vi "CalcIMUBias.vi"(10 "error in (no error)":errorcluster) -> (1 "Bias":T1, 3 "error out":errorcluster)   [LabVIEW 2016]
uses:
  <vilib>/Platform/TimedLoop/XDataNode/timing_clust.ctl
  <vilib>/Platform/TimedLoop/XDataNode/nitl_modes.ctl
  <vilib>/Platform/TimedLoop/XDataNode/wakeup.ctl
  <vilib>/Platform/TimedLoop/XDataNode/XDataNode.xnode
  <vilib>/Platform/TimedLoop/XDataNode/XDNodeRunTimeDep.lvlib
panel:
  out "Z gyro bias":dbl
  out "Y gyro bias":dbl
  out "X gyro bias":dbl
  out "Z acc bias":dbl
  out "Y acc bias":dbl
  out "X acc bias":dbl
  out "Accel, Gyro":u16[](array[numeric])
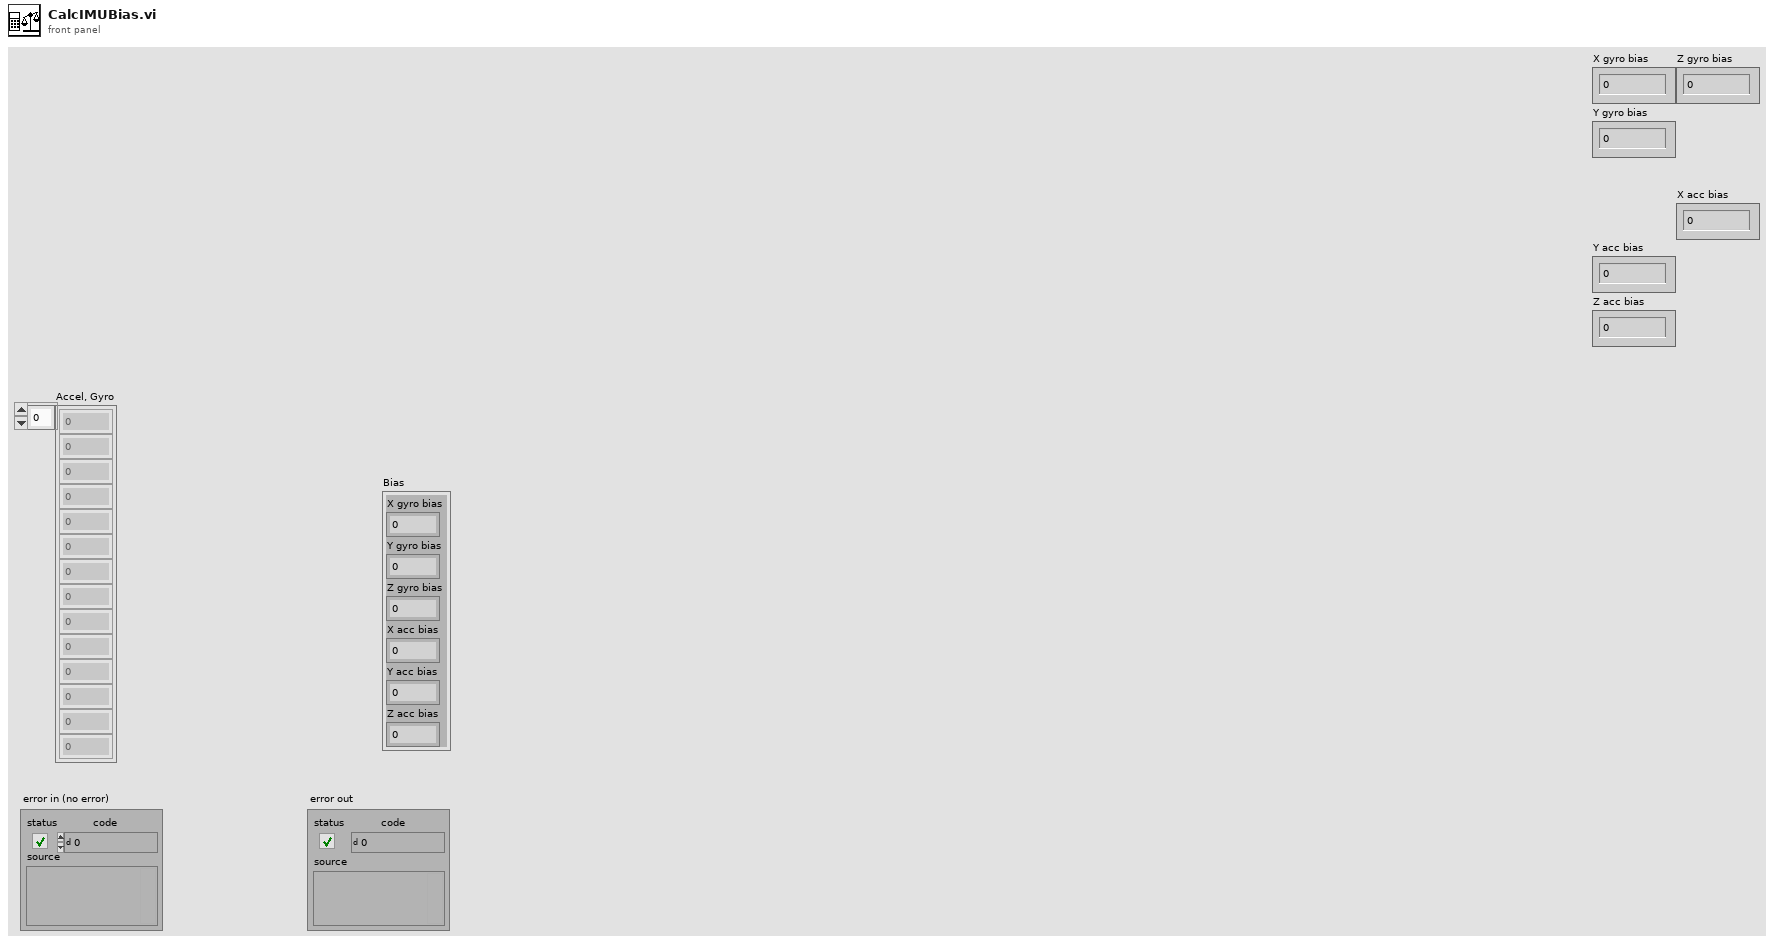
[diagram p1: front panel]
types:
  T1 = cluster{"X gyro bias":dbl, "Y gyro bias":dbl, "Z gyro bias":dbl, "X acc bias":dbl, "Y acc bias":dbl, "Z acc bias":dbl}
  T2 = typedef "XDNodeRunTimeDep.lvlib/timing_clust.ctl" = cluster{"Expected End [f-1]":u64, "Actual End [f-1]":u64, "Finished Late? [f-1]":bool, "Expected End [i-1]":u64, "Actual End [i-1]":u64, "Finished Late? [i-1]":bool, "Expected Start [i]":u64, "Actual Start [i]":u64, "Expected Start [f]":u64, "Actual Start [f]":u64, "Source Name":string, "Structure Name":string, "Period":i64, "Deadline":i64, "Offset":i64, "Start":i64, "Priority":i32, "Timeout":i32, "Mode":T3, "Wakeup Reason":T4, "Error":errorcluster, "Source Type":string, "Secondary Source Type":string, "Global End Time":u64, "Global Start Time":u64, "Frame Duration":u64, "Iteration Duration":u64, "Assigned CPU":i32, "I/O Scan Engine Mode":u32}
  T3 = typedef "XDNodeRunTimeDep.lvlib/nitl_modes.ctl" = enum32{"No Change", "Process missed periods, maintain original phase", "Discard missed periods, maintain original phase", "Process missed periods, ignore original phase", "Discard missed periods, ignore original phase"}
  T4 = typedef "XDNodeRunTimeDep.lvlib/wakeup.ctl" = enum32{"Normal", "Aborted", "Asynchronous wakeup", "Timing source error", "Timed loop error", "Timeout"}
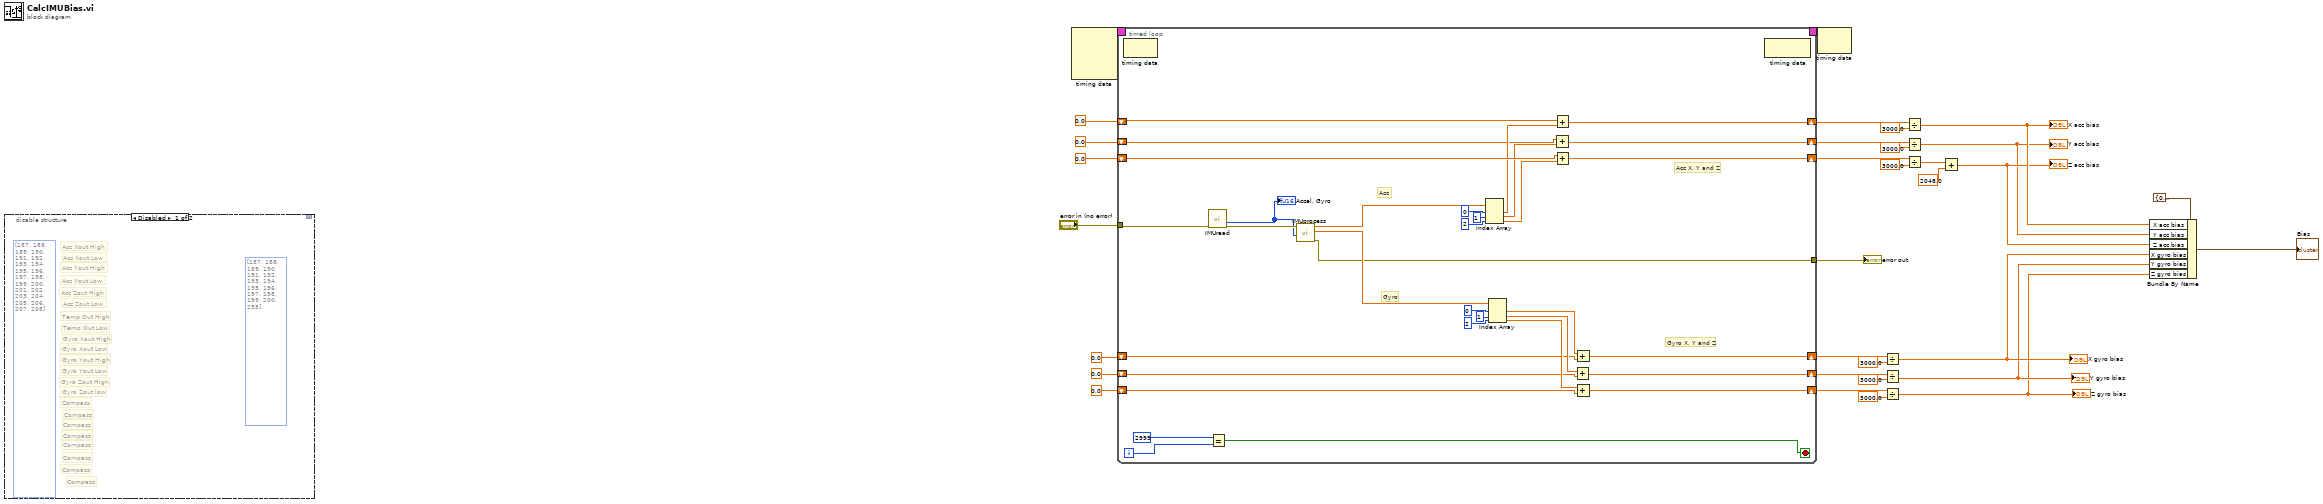
[diagram p0: block diagram]
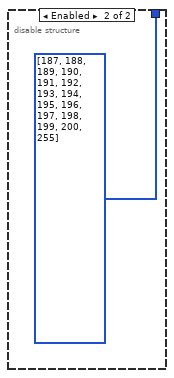
[diagram p2: hidden frame]
diagram:
  n1 = disable-structure shown="Disabled" {
    disable-tunnel: [_ u16[] [187, 188, 189, 190, 191, 192, 193, 194, 195, 196, 197, 198, 199, 200, 255] ("Frames to Write")] -> _
    frame Disabled {
      (unwired) u16[] [187, 188, 189, 190, 191, 192, 193, 194, 195, 196, 197, 198, 199, 200, 201, 202, 203, 204, 205, 206, 207, 208] ("Frames to Write")
      (unwired) u16[] [187, 188, 189, 190, 191, 192, 193, 194, 195, 196, 197, 198, 199, 200, 255] ("Frames to Write")
      # "Compass"
      # "Compass"
      # "Compass"
      # "Compass"
      # "Compass"
      # "Compass"
      # "Compass"
      # "Compass"
      # "Gyro Zout low"
      # "Gyro Zout High"
      # "Gyro Yout Low"
      # "Gyro Yout High"
      # "Gyro Xout Low"
      # "Gyro Xout High"
      # "Temp Out Low"
      # "Temp Out High"
      # "Acc Zout Low"
      # "Acc Zout High"
      # "Acc Yout Low"
      # "Acc Yout High"
      # "Acc Xout Low"
      # "Acc Xout High"
    }
    frame Enabled {
    }
  }
  n2 = node-c288() -> (w32:T2)  [unwired: 4 in]
  n3 = timed-loop {
    timing: w32 -> [_]
    timing-out: [_] -> w31
    shift-right: [w56] -> w22
    shift-left: 0.0 -> [w58]
    shift-right: [w55] -> w21
    shift-left: 0.0 -> [w52]
    shift-right: [w54] -> w20
    shift-left: 0.0 -> [w57]
    tunnel: [w49] -> w27
    tunnel: "error in (no error)" -> [w48]
    shift-right: [w47] -> w15
    shift-left: 0.0 -> [w41]
    shift-right: [w46] -> w14
    shift-left: 0.0 -> [w40]
    shift-right: [w45] -> w13
    shift-left: 0.0 -> [w39]
    i -> [w38]
    stop <- w36 stop-if-true
    # "Gyro"
    # "Acc"
    # "Gyro X, Y and Z"
    # "Acc X, Y and Z"
    n4 = node-c288() -> ()  [unwired: 1 in, 1 out]
    n5 = call "IMUread.vi"("error in (no error)"=w48) -> ("error out"=w66:errorcluster, "Accel, Gyro"=w35:u16[])  [unwired: 9 in]
    "Accel, Gyro" <- w35
    n6 = Equal?(x=2999, y=w38) -> (x = y?=w36:bool)
    n7 = call "IMUprocess.vi"("Frames Read"=w35, "error in (no error)"=w66) -> ("error out"=w49:errorcluster, "Gyro deg/s"=w63:dbl[], "Accel g's"=w34:dbl[])  [unwired: 7 in]
    n8 = Index Array(array=w34, index #1=0 ("index"), index #2=1 ("index"), index #3=2 ("index")) -> (element #1=w53:dbl, element #2=w51:dbl, element #3=w50:dbl)
    n9 = Index Array(array=w63, index #1=0 ("index"), index #2=1 ("index"), index #3=2 ("index")) -> (element #1=w44:dbl, element #2=w43:dbl, element #3=w42:dbl)
    n10 = Add(x=w52, y=w51) -> (x+y=w55:dbl)
    n11 = Add(x=w58, y=w53) -> (x+y=w56:dbl)
    n12 = Add(x=w57, y=w50) -> (x+y=w54:dbl)
    n13 = Add(x=w43, y=w40) -> (x+y=w46:dbl)
    n14 = Add(x=w44, y=w41) -> (x+y=w47:dbl)
    n15 = Add(x=w42, y=w39) -> (x+y=w45:dbl)
    n16 = node-c288() -> ()  [unwired: 1 in, 1 out]
  }
  "error out" <- w27
  n17 = node-c288(w31) -> ()  [unwired: 1 out]
  n18 = Divide(x=w15, y=3000.0) -> (x/y=w10:dbl)
  "X gyro bias" <- w10
  n19 = Divide(x=w14, y=3000.0) -> (x/y=w9:dbl)
  "Y gyro bias" <- w9
  n20 = Divide(x=w13, y=3000.0) -> (x/y=w8:dbl)
  "Z gyro bias" <- w8
  n21 = Divide(x=w22, y=3000.0) -> (x/y=w7:dbl)
  "X acc bias" <- w7
  n22 = Divide(x=w21, y=3000.0) -> (x/y=w1:dbl)
  "Y acc bias" <- w1
  n23 = Divide(x=w20, y=3000.0) -> (x/y=w4:dbl)
  n24 = Add(x=w4, y=2048.0) -> (x+y=w3:dbl)
  "Z acc bias" <- w3
  n25 = Bundle By Name(cluster=T1 {"X gyro bias"=0.0, "Y gyro bias"=0.0, "Z gyro bias"=0.0, "X acc bias"=0.0, "Y acc bias"=0.0, "Z acc bias"=0.0} ("Cluster"), "X acc bias"=w7, "Y acc bias"=w1, "Z acc bias"=w3, "X gyro bias"=w10, "Y gyro bias"=w9, "Z gyro bias"=w8) -> (→"Bias":T1)
